vi "Precio VS Credito.vi"(8 "error in (no error)":errorcluster, 10 "Cluster Producto":T1, 11 "USD Actor in":refnum<class "USD Actor.lvclass">) -> (0 "error out":errorcluster, 3 "USD Actor out":refnum<class "USD Actor.lvclass">)   [LabVIEW 2019, in "USD Actor.lvlib" / "USD Actor.lvclass"]
uses:
  USD Actor.lvclass
  C:/Program Files (x86)/National Instruments/LabVIEW 2019/vi.lib/ActorFramework/Actor/Actor.lvclass
  5 SEMESTRE/INTERFACES/Ejer_labview/Maquina_Expendedora/Control 1.ctl
  <vilib>/ActorFramework/Actor/Actor.lvclass/Actor.ctl
  USD Actor.lvclass/USD Actor.ctl
  UI Actor Messages/Actualizar Estatus Msg/Actualizar Estatus Msg.lvclass/Actualizar Estatus Msg.ctl
  <vilib>/ActorFramework/Message Enqueuer/Message Enqueuer.lvclass/Message Enqueuer.ctl
  <vilib>/ActorFramework/Message Enqueuer/Enqueue.vi
  UI Actor Messages/Actualizar Estatus Msg/Actualizar Estatus Msg.lvclass
  C:/Program Files (x86)/National Instruments/LabVIEW 2019/vi.lib/ActorFramework/Message/Message.lvclass
  <vilib>/ActorFramework/Message Priority Queue/Priority Enqueue.vi
  CAFE ACTOR/CAFE ACTOR.lvclass
  REFRESCOS Y PAPAS ACTOR/REFRESCOS Y PAPAS ACTOR.lvclass
  <vilib>/ActorFramework/Actor/Actor.lvclass
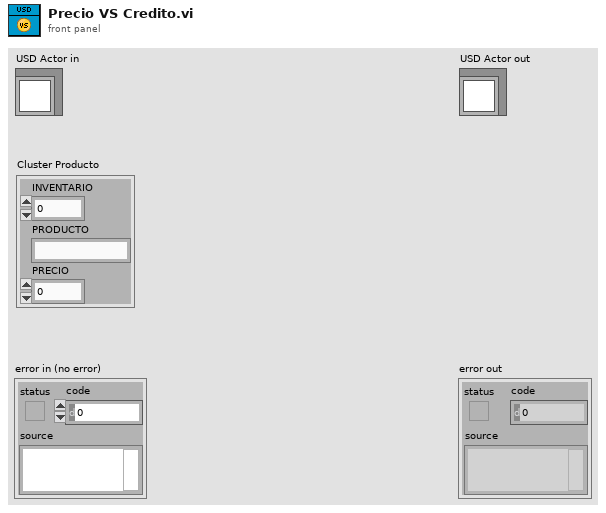
[diagram p1: front panel]
types:
  T1 = cluster{"INVENTARIO":i32, "PRODUCTO":string, "PRECIO":dbl}
  T2 = typedef "Control 1.ctl" = u16
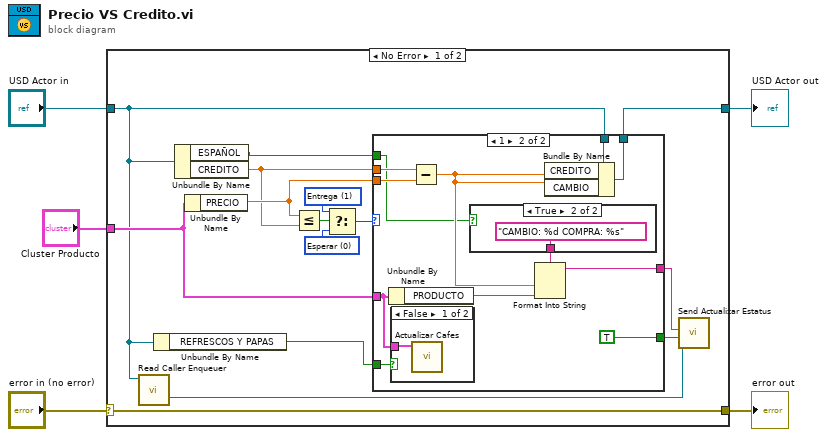
[diagram p0: block diagram]
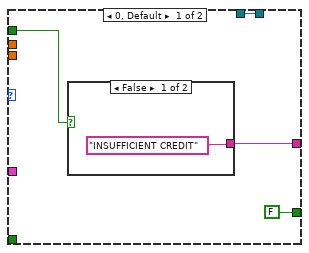
[diagram p2: hidden frame]
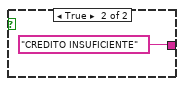
[diagram p3: hidden frame]
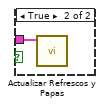
[diagram p4: hidden frame]
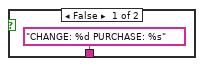
[diagram p5: hidden frame]
diagram:
  n1 = case shown="No Error" "error in (no error)" {
    selector: "error in (no error)" -> [w20 w44]
    tunnel: [w20 w44] -> w3
    tunnel: [w13 w43] -> w2
    tunnel: "USD Actor in" -> [w9 w43]
    tunnel: "Cluster Producto" -> [w15 _]
    frame No Error {
      w16 = T2 0 items=["Esperar", "Entrega"] ("Estados")
      w19 = T2 1 items=["Esperar", "Entrega"] ("Estados")
      n2 = call <vilib>:"Read Caller Enqueuer.vi"("Actor"=w9) -> ("Caller Enqueuer"=w6:refnum<class "Message Enqueuer.lvclass">)  [unwired: 10 in]
      n3 = Unbundle By Name(w9) -> ("REFRESCOS Y PAPAS"=w11:bool)
      n4 = Unbundle By Name(w9) -> ("ESPAÑOL"=w12:bool, "CREDITO"=w10:dbl)
      n5 = Unbundle By Name(w15) -> ("PRECIO"=w14:dbl)
      n6 = Less Or Equal?(x=w14, y=w10) -> (x <= y?=w18:bool)
      n7 = Select(t=w19, s=w18, f=w16) -> (s? t:f=w17:T2)
      n8 = case shown="1" w17 {
        tunnel: w9 -> [w24 w38]
        tunnel: [w24 w37] -> w13
        tunnel: w15 -> [_ w30]
        tunnel: w10 -> [_ w33]
        tunnel: w14 -> [_ w32]
        tunnel: w12 -> [w23 w31]
        tunnel: w11 -> [_ w29]
        tunnel: [w22 w28] -> w8
        tunnel: [FALSE TRUE] -> w7
        frame 0, Default {
          n9 = case shown="False" w23 {
            tunnel: ["INSUFFICIENT CREDIT" ("Message") "CREDITO INSUFICIENTE" ("Message")] -> w22
            frame False {
            }
            frame True {
            }
          }
        }
        frame 1 {
          n10 = Unbundle By Name(w30) -> ("PRODUCTO"=w36:string)
          n11 = case shown="False" w29 {
            tunnel: w30 -> [w39 w40]
            frame False {
              n12 = call "Actualizar Cafes.vi"("Cluster Producto"=w39) -> ()  [unwired: 11 in]
            }
            frame True {
              n13 = call "Actualizar Refrescos y Papas.vi"("Cluster Producto"=w40) -> ()  [unwired: 11 in]
            }
          }
          n14 = Subtract(x=w33, y=w32) -> (x-y=w35:dbl)
          n15 = case shown="True" w31 {
            tunnel: ["CHANGE: %d PURCHASE: %s" ("format string") "CAMBIO: %d COMPRA: %s" ("format string")] -> w34
            frame False {
            }
            frame True {
            }
          }
          n16 = Format Into String(format string=w34, w35, w36) -> (resulting string=w28:string)  [unwired: 2 in, 1 out]
          n17 = Bundle By Name(cluster=w38, "CREDITO"=w35, "CAMBIO"=w35) -> (w37:refnum<class "USD Actor.lvclass">)
        }
      }
      n18 = call "Send Actualizar Estatus.vi"("ACTUALIZA TABLA"=w7, "ESTATUS"=w8, "Message Enqueuer"=w6) -> ()  [unwired: 7 in, 2 out]
    }
    frame Error {
    }
  }
  "error out" <- w3
  "USD Actor out" <- w2
